vi "停止命令.vi"(7 "是否启用通讯通知":bool, 8 "error in (no error)":errorcluster, 11 "Slave ID":T1) -> (0 "error out":errorcluster)   [LabVIEW 2016, in "质控单元V1.lvlib"]
uses:
  <vilib>/Plasmionique/MB Master/MB_Master/MB_Master.lvclass
  <vilib>/Plasmionique/MB Master/MB Master.lvlib
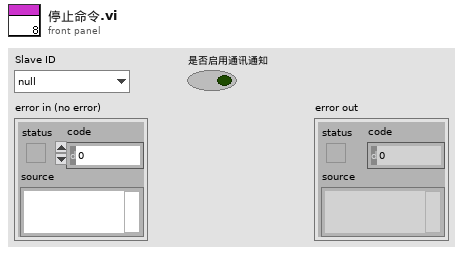
[diagram p1: front panel]
types:
  T1 = typedef "质控单元V1.lvlib/质控slave id.ctl" = enum16{"null", "氨氮", "总磷", "CODMn", "CODCr", "总氮"}
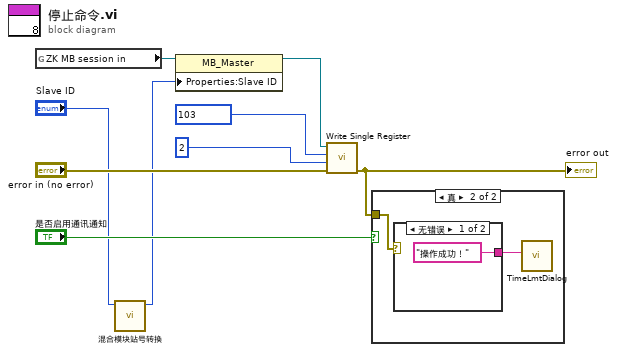
[diagram p0: block diagram]
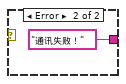
[diagram p3: hidden frame]
diagram:
  n1 = global read "ZK非断电保存全局变量.vi" "ZK MB session in"() -> (w8:refnum<class "MB_Master.lvclass">)
  n2 = call "混合模块站号转换.vi"("Slave ID输入"="Slave ID") -> ("Slave ID输出"=w1:T1)  [unwired: 10 in]
  n3 = property class="MB_Master"(reference=w8, "Properties:Slave ID"=w1) -> (reference out=w6:refnum<class "MB_Master.lvclass">)  [unwired: 1 in, 1 out]
  n4 = call <vilib>:"Write Single Register.vi"("error in (no error)"="error in (no error)", "value"=u16 2, "address"=u16 103 ("starting address"), "MB session in"=w6) -> ("error out"=w4:errorcluster)  [unwired: 6 in, 1 out]
  "error out" <- w4
  n5 = case shown="真" "是否启用通讯通知" {
    tunnel: w4 -> [_ w11]
    frame False {
    }
    frame True {
      n6 = case shown="无错误" w11 {
        tunnel: ["操作成功！" "通讯失败！"] -> w10
        frame No Error {
        }
        frame Error {
        }
      }
      n7 = call "TimeLmtDialog.vi"("Infoin"=w10) -> ()  [unwired: 11 in]
    }
  }
